vi "Is schedule empty.vi"(8 "error in (no error)":errorcluster, 11 "Run Block in":refnum<class "Run Block.lvclass">) -> (0 "error out":errorcluster, 1 "Schedule out":refnum<class "Schedule.lvclass">, 2 "Empty?":bool, 3 "Run Block out":refnum<class "Run Block.lvclass">)   [LabVIEW 2020, in "TALOS.lvlib" / "Run Utilities.lvlib" / "Run Block.lvclass"]
doc: "Checks whether the schedule is empty. Returns current schedule along the indicator"
uses:
  Run Block.lvclass
  Schedule/Schedule.lvclass
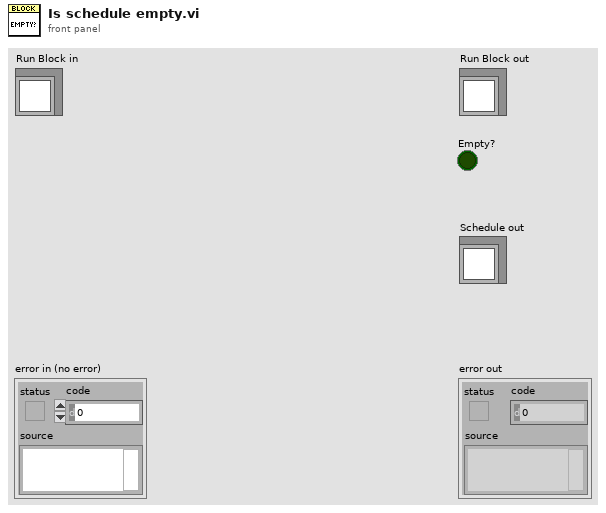
[diagram p1: front panel]
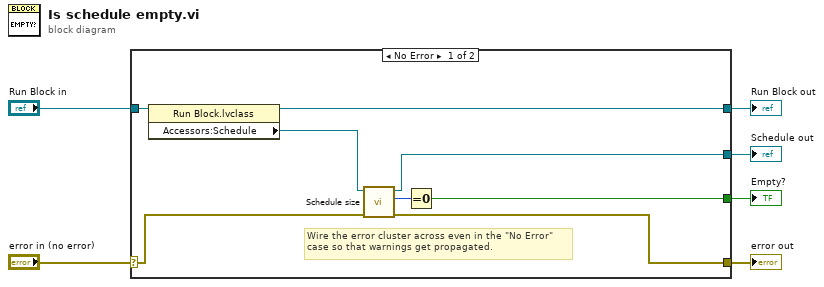
[diagram p0: block diagram]
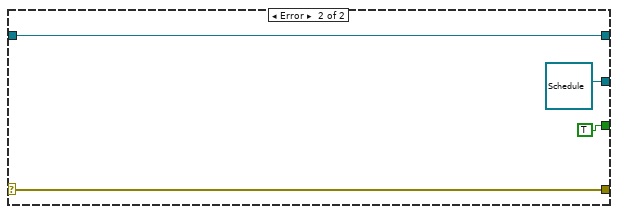
[diagram p2: hidden frame]
diagram:
  n1 = case shown="No Error" "error in (no error)" {
    selector: "error in (no error)" -> [w11 w18]
    tunnel: [w10 w18] -> w5
    tunnel: [w13 w17] -> w3
    tunnel: "Run Block in" -> [w14 w17]
    tunnel: [w8 TRUE] -> w1
    tunnel: [w7 refnum<class "Schedule.lvclass"> refnum ("Schedule out")] -> w2
    frame No Error {
      # "Wire the error cluster across even in the \"No Error\"\ncase so that warnings get propagated."
      n2 = property class="Run Block.lvclass"(reference=w14) -> (reference out=w13:refnum<class "Run Block.lvclass">, "Accessors:Schedule"=w12:refnum<class "Schedule.lvclass">)  [unwired: 1 in, 1 out]
      n3 = call-dynamic "Schedule size.vi"("error in (no error)"=w11, "Schedule in"=w12) -> ("error out"=w10:errorcluster, "Size"=w9:i32, "Schedule out"=w7:refnum<class "Schedule.lvclass">)  [unwired: 7 in]
      n4 = Equal To 0?(x=w9) -> (x = 0?=w8:bool)
    }
    frame Error {
    }
  }
  "error out" <- w5
  "Run Block out" <- w3
  "Schedule out" <- w2
  "Empty?" <- w1
